vi "ProjectOpen.vi"(6 "Visible?":bool, 7 "Sequence Context":refnum<k7>, 8 "password":string, 9 "username":string, 10 "Project File Path":path, 11 "Gateway IP Address (\"\": localhost)":string) -> (0 "error out":errorcluster)   [LabVIEW 2015, in "ni-veristand-steps-runtime-lib.lvlib"]
uses:
  ni-veristand-steps-runtime-lib.lvlib
  NationalInstruments.VeriStand.ClientAPI
  <vilib>/NI Veristand/Execution/Project/NI_VS Project ExecutionAPI.lvlib
panel:
  in  "error in (no error)":errorcluster
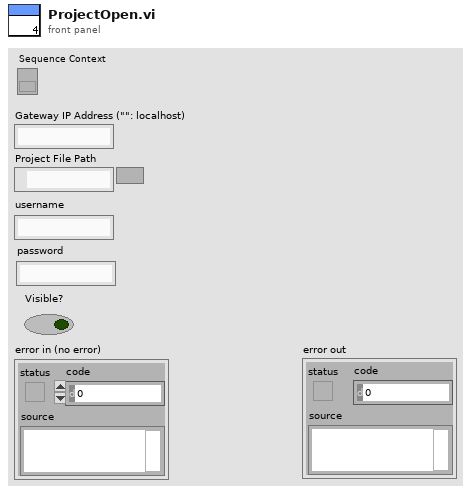
[diagram p1: front panel]
types:
  T1 = typedef "ni-veristand-steps-runtime-lib.lvlib/VeriStand dotNet References.ctl" = cluster{"Project Ref":refnum<k24>, "Workspace Manager Ref":refnum<k24>, "Model Manager Ref":refnum<k24>, "Channel Fault Manager Ref":refnum<k24>}
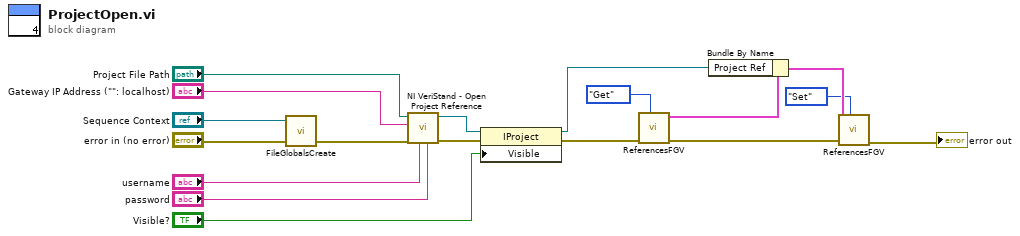
[diagram p0: block diagram]
diagram:
  n1 = call "FileGlobalsCreate.vi"("error in (no error)"="error in (no error)", "Sequence Context"="Sequence Context") -> ("error out"=w12:errorcluster)  [unwired: 3 in]
  n2 = call <vilib>:"NI VeriStand - Open Project Reference.vi"("Password"="password", "Username"="username", "error in (no error)"=w12, "Gateway IP Address (\"\": localhost)"="Gateway IP Address (\"\": localhost)", "Project File Path"="Project File Path") -> ("error out"=w10:errorcluster, "Project Ref"=w11:refnum<k24>)  [unwired: 5 in]
  n3 = property class="IProject"(reference=w11, error in=w10, "Visible"="Visible?") -> (reference out=w6:refnum<k24>, error out=w3:errorcluster)
  n4 = call "ReferencesFGV.vi"("Get/Set"=enum16{"Get", "Set"}."Get", "error in (no error)"=w3) -> ("error out"=w2:errorcluster, "VeriStand dotNET Refs out"=w1:T1)  [unwired: 8 in]
  n5 = Bundle By Name(cluster=w1, "Project Ref"=w6) -> (w8:T1)
  n6 = call "ReferencesFGV.vi"("Get/Set"=enum16{"Get", "Set"}."Set", "error in (no error)"=w2, "VeriStand dotNET Refs"=w8) -> ("error out"=→"error out":errorcluster)  [unwired: 7 in, 1 out]
